vi "Press And Hold Button .vi"(0 "GEA2 Reference In":refnum<k24>, 1 "Delay Time (s)":dbl=3.25 format="%#_13g", 5 "Standalone?":bool, 7 "Button":T2=enum."SW201 - My Cycle", 9 "GEA Inputs":T1 {"Destination" format="%.0x"; "Source" format="%.0x"}, 11 "Error In":errorcluster) -> (4 "GEA2 Reference Out":refnum<k24>, 15 "Error Out":errorcluster)   [LabVIEW 2018, in "TLMB.lvlib"]
uses:
  Projects/TLMB.lvlib
  type defs/UI Buttons.ctl
  D:/Common/LabVIEW GEA2 Toolkit/source/GEA3 DLL Source/GeaCommunication.dll
  Common/LabVIEW GEA2 Toolkit/source/GEA3 DLL Source/GeaCommunication.dll
  Common/LabVIEW GEA2 Toolkit/GEA3/type defs/Source_Destination.ctl
  Common/LabVIEW GEA2 Toolkit/GEA3/type defs/ERD Write Data In.ctl
  Common/LabVIEW GEA2 Toolkit/GEA3/type defs/Data Type.ctl
  C:/Users/iallatyp/Desktop/New folder/GEA3/library/GEA2_Toolkit.lvlib
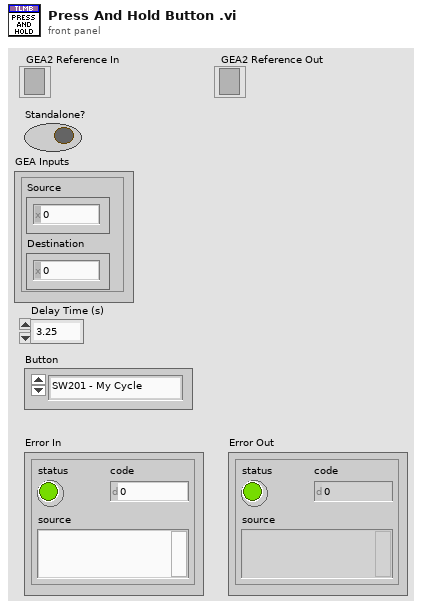
[diagram p1: front panel]
types:
  T1 = typedef "GEA2_Toolkit.lvlib/Source_Destination.ctl" = cluster{"Source":u8, "Destination":u8}
  T2 = typedef "TLMB.lvlib/UI Buttons.ctl" = enum16{"Switch Off", "SW201 - My Cycle", "SW202 - Delay Wash", "SW203 - Extra Rinse", "SW204 - Signal / Volume", "SW205 - Spin", "SW206 - Deep Rinse / Fab Soft", "SW207 - Soil", "SW208 - Auto Soak", "SW209 - Temp", "SW210 - Warm Rinse", "SW211 - Deep Fill", "SW212 - Stain Remover", "SW213 - Power", "SW222 - Control Lock", "SW214 - Start / Pause", "SW301 - Start/Pause LE", "SW302 - Option Button LE", "SW201/212 - Bulk Flush"}
  T3 = typedef "GEA2_Toolkit.lvlib/ERD Write Data In.ctl" = cluster{"ERD Number":u16, "Data Type":T4, "Data":string}
  T4 = typedef "GEA2_Toolkit.lvlib/Data Type.ctl" = enum16{"string", "boolean", "uint8_t", "uint16_t", "uint32_t", "uint64_t", "int8_t", "int16_t", "int32_t", "int64_t"}
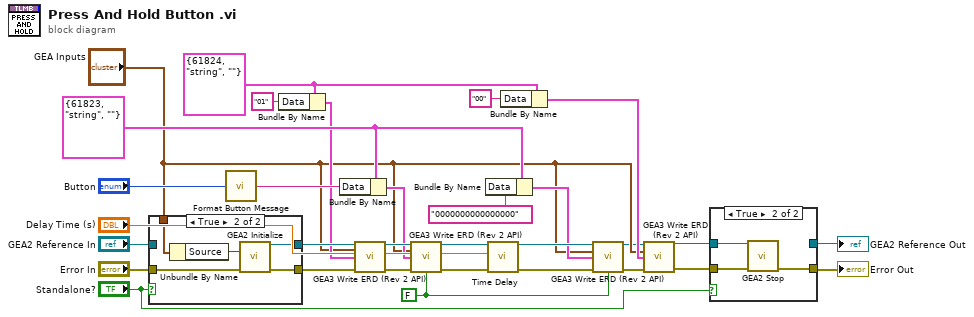
[diagram p0: block diagram]
diagram:
  w8 = T3 {"ERD Number"=61824, "Data Type"=enum."string", "Data"=""} ("ERD Write Data In")
  w11 = FALSE ("Verify ERD Response?")
  w22 = T3 {"ERD Number"=61823, "Data Type"=enum."string", "Data"=""} ("ERD Write Data In")
  n1 = case shown="True" "Standalone?" {
    tunnel: "Error In" -> [w31 w37]
    tunnel: [w31 w36] -> w20
    tunnel: "GEA2 Reference In" -> [w32 _]
    tunnel: [w32 w35] -> w21
    tunnel: "GEA Inputs" -> [_ w33]
    frame False {
    }
    frame True {
      n2 = Unbundle By Name(w33) -> ("Source"=w34:u8)
      n3 = call "GEA2 Initialize.vi"("Source Address"=w34, "error in"=w37) -> ("GEA2 Reference Out"=w35:refnum<k24>, "error out"=w36:errorcluster)  [unwired: 11 in, 1 out]
    }
  }
  n4 = call "Format Button Message.vi"("Switch"="Button") -> ("Switch Message"=w24:string)  [unwired: 14 in]
  n5 = Bundle By Name(cluster=w8, "Data"="01") -> (w18:T3)
  n6 = Bundle By Name(cluster=w22, "Data"=w24) -> (w10:T3)
  n7 = call "GEA3 Write ERD (Rev 2 API).vi"("GEA2 Reference In"=w21, "GEA Inputs"="GEA Inputs", "ERD Write Data In"=w18, "Error In"=w20) -> ("GEA2 Reference Out"=w17:refnum<k24>, "Error Out"=w16:errorcluster)  [unwired: 9 in, 1 out]
  n8 = call "GEA3 Write ERD (Rev 2 API).vi"("GEA2 Reference In"=w17, "GEA Inputs"="GEA Inputs", "ERD Write Data In"=w10, "Error In"=w16, "Verify ERD Response?"=w11) -> ("GEA2 Reference Out"=w14:refnum<k24>, "Error Out"=w15:errorcluster)  [unwired: 8 in, 1 out]
  n9 = Bundle By Name(cluster=w22, "Data"="0000000000000000" ("Message")) -> (w12:T3)
  n10 = call "Time Delay"("error in (no error)"=w15, "Delay Time (s)"="Delay Time (s)") -> ("error out"=w13:errorcluster)  [unwired: 9 in]
  n11 = Bundle By Name(cluster=w8, "Data"="00") -> (w6:T3)
  n12 = call "GEA3 Write ERD (Rev 2 API).vi"("GEA2 Reference In"=w14, "GEA Inputs"="GEA Inputs", "ERD Write Data In"=w12, "Error In"=w13, "Verify ERD Response?"=w11) -> ("GEA2 Reference Out"=w4:refnum<k24>, "Error Out"=w9:errorcluster)  [unwired: 8 in, 1 out]
  n13 = call "GEA3 Write ERD (Rev 2 API).vi"("GEA2 Reference In"=w4, "GEA Inputs"="GEA Inputs", "ERD Write Data In"=w6, "Error In"=w9) -> ("GEA2 Reference Out"=w3:refnum<k24>, "Error Out"=w2:errorcluster)  [unwired: 9 in, 1 out]
  n14 = case shown="True" "Standalone?" {
    tunnel: [w39 w42] -> w26
    tunnel: w3 -> [w38 w41]
    tunnel: w2 -> [w39 w40]
    tunnel: [w38 _] -> w1
    frame False {
    }
    frame True {
      n15 = call "GEA2 Stop.vi"("GEA2 Reference In"=w41, "Error In"=w40) -> ("Error Out"=w42:errorcluster)  [unwired: 13 in]
    }
  }
  "Error Out" <- w26
  "GEA2 Reference Out" <- w1
